vi "Check Cluster Term Type.vi"(8 "Error In (no Error) In":errorcluster, 10 "Element Check In":T1(ring), 11 "Term Type In":T2) -> (0 "Error Out":errorcluster, 3 "Is Good ?":bool, 5 "Elements":i32)   [LabVIEW 2012, in "Scripting Tools.lvlib" / "XNode Support.lvlib"]
doc: "Inspect a terminal to see if it is a cluster with certain characteristics (e.g. all elements the same type, all numeric, all sortable etc)."
uses:
  XNode Support.lvlib
  <vilib>/XNodeSupport/XNodeTermTypeIDPair.ctl
  <vilib>/XNodeSupport/XNodeType.ctl
  <vilib>/XNodeSupport/XNodeString.ctl
  <vilib>/Utility/VariantDataType/VariantType.lvlib
  <vilib>/XNodeSupport/NI_XNodeSupport.lvlib
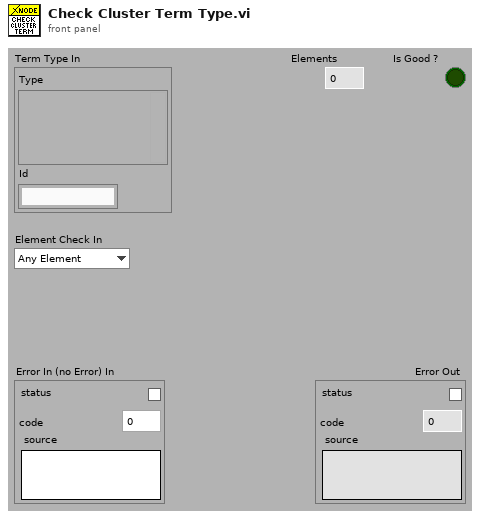
[diagram p1: front panel]
types:
  T1 = enum16{"Any Element", "All Numeric", "All Integer", "All Float", "All Complex", "All Sortable", "Error Cluster", "All the same type"}
  T2 = typedef "NI_XNodeSupport.lvlib/XNodeTermTypeIDPair.ctl" = cluster{"Type":T3, "Id":T4}
  T3 = typedef "NI_XNodeSupport.lvlib/XNodeType.ctl" = variant
  T4 = typedef "NI_XNodeSupport.lvlib/XNodeString.ctl" = string
  T5 = typedef "VariantType.lvlib/Type.ctl" = enum8{"Invalid Type", "Void", "I8", "I16", "I32", "I64", "U8", "U16", "U32", "U64", "Single Float", "Double Float", "Extended Float", "Single Complex", "Double Complex", "Extended Complex", "Enum U8", "Enum U16", "Enum U32", "Enum U64", "Single Float With Unit", "Double Float With Unit", "Extended Float With Unit", "Single Complex with Unit", "Double Complex with Unit", "Extended Complex with Unit", "Boolean", "String", "Path", "Picture", "Tag", "Array", "Cluster", "Variant", "LV Variant", "Waveform", "Timestamp", "Digital Waveform", "Digital Data", "ExpressData", "Refnum", "External Data", "VI", "Poly VI", "LabVIEW Class Instance", "Fixed Point"}
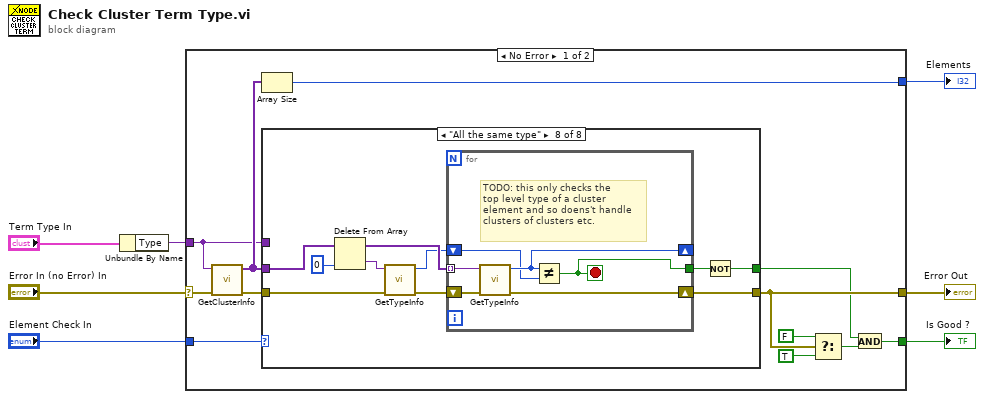
[diagram p0: block diagram]
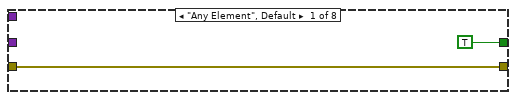
[diagram p2: hidden frame]
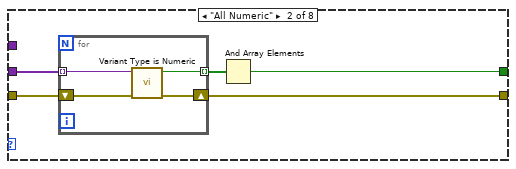
[diagram p3: hidden frame]
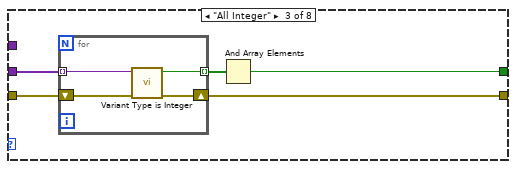
[diagram p4: hidden frame]
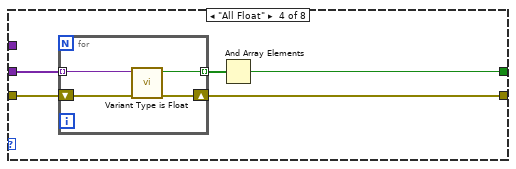
[diagram p5: hidden frame]
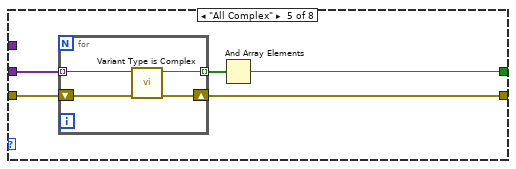
[diagram p6: hidden frame]
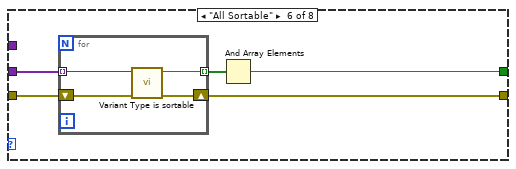
[diagram p7: hidden frame]
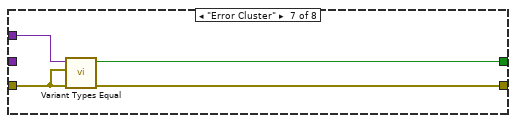
[diagram p8: hidden frame]
diagram:
  n1 = Unbundle By Name("Term Type In") -> ("Type"=w5:T3)
  n2 = case shown="No Error" "Error In (no Error) In" {
    selector: "Error In (no Error) In" -> [w19 w87]
    tunnel: w5 -> [w9 _]
    tunnel: [w18 _] -> w4
    tunnel: "Element Check In" -> [w17 _]
    tunnel: [w15 w87] -> w2
    tunnel: [w11 _] -> w1
    frame No Error {
      n3 = call <vilib>:"GetClusterInfo.vi"("error in (no error)"=w19, "Variant"=w9) -> ("error out"=w16:errorcluster, "Cluster Elements"=w10:variant[])  [unwired: 8 out]
      n4 = Array Size(array=w10) -> (size(s)=w18:i32)
      n5 = case shown="\"All the same type\"" w17 {
        tunnel: w16 -> [w21 w26 w35 w44 w53 w62 w70 w76]
        tunnel: [w21 w25 w34 w43 w52 w61 w68 w73] -> w15
        tunnel: [TRUE w24 w33 w42 w51 w60 w67 w71] -> w12
        tunnel: w10 -> [_ w23 w32 w41 w50 w59 _ w80]
        tunnel: w9 -> [_ _ _ _ _ _ w69 _]
        frame "Any Element", Default {
        }
        frame "All Numeric" {
          n6 = for {
            shift-right: [w27] -> w25
            shift-left: w26 -> [w30]
            tunnel: w23 -> [w29] mode=indexing
            tunnel: [w28] -> w22 mode=indexing
            n7 = call "Variant Type is Numeric.vi"("error in (no error)"=w30, "Type"=w29) -> ("error out"=w27:errorcluster, "Sortable ?"=w28:bool)  [unwired: 8 out]
          }
          n8 = And Array Elements(Boolean array=w22) -> (logical AND=w24:bool)
        }
        frame "All Integer" {
          n9 = for {
            shift-right: [w36] -> w34
            shift-left: w35 -> [w39]
            tunnel: w32 -> [w38] mode=indexing
            tunnel: [w37] -> w31 mode=indexing
            n10 = call "Variant Type is Integer.vi"("error in (no error)"=w39, "Type"=w38) -> ("error out"=w36:errorcluster, "Sortable ?"=w37:bool)  [unwired: 8 out]
          }
          n11 = And Array Elements(Boolean array=w31) -> (logical AND=w33:bool)
        }
        frame "All Float" {
          n12 = for {
            shift-right: [w45] -> w43
            shift-left: w44 -> [w48]
            tunnel: w41 -> [w47] mode=indexing
            tunnel: [w46] -> w40 mode=indexing
            n13 = call "Variant Type is Float.vi"("error in (no error)"=w48, "Type"=w47) -> ("error out"=w45:errorcluster, "Sortable ?"=w46:bool)  [unwired: 8 out]
          }
          n14 = And Array Elements(Boolean array=w40) -> (logical AND=w42:bool)
        }
        frame "All Complex" {
          n15 = for {
            shift-right: [w54] -> w52
            shift-left: w53 -> [w57]
            tunnel: w50 -> [w56] mode=indexing
            tunnel: [w55] -> w49 mode=indexing
            n16 = call "Variant Type is Complex.vi"("error in (no error)"=w57, "Type"=w56) -> ("error out"=w54:errorcluster, "Sortable ?"=w55:bool)  [unwired: 8 out]
          }
          n17 = And Array Elements(Boolean array=w49) -> (logical AND=w51:bool)
        }
        frame "All Sortable" {
          n18 = for {
            shift-right: [w63] -> w61
            shift-left: w62 -> [w66]
            tunnel: w59 -> [w65] mode=indexing
            tunnel: [w64] -> w58 mode=indexing
            n19 = call "Variant Type is sortable.vi"("error in (no error)"=w66, "Type"=w65) -> ("error out"=w63:errorcluster, "Sortable ?"=w64:bool)  [unwired: 8 out]
          }
          n20 = And Array Elements(Boolean array=w58) -> (logical AND=w60:bool)
        }
        frame "Error Cluster" {
          n21 = call "Variant Types Equal.vi"("error in (no error)"=w70, "Type"=w70, "Type to Test"=w69) -> ("error out"=w68:errorcluster, "Same Type"=w67:bool)  [unwired: 7 out]
        }
        frame "All the same type" {
          n22 = Delete From Array(array=w80, index=0) -> (deleted portion=w77:variant, array with subset deleted=w79:variant[])  [unwired: 1 in]
          n23 = call <vilib>:"GetTypeInfo.vi"("error in (no error)"=w76, "Variant"=w77) -> ("error out"=w75:errorcluster, "Type Enum"=w74:T5)  [unwired: 8 out]
          n24 = for {
            tunnel: w79 -> [w86] mode=indexing
            shift-right: [w82] -> w73
            shift-left: w75 -> [w85]
            shift-right: [w84] -> _
            shift-left: w74 -> [w83]
            tunnel: [w81] -> w72
            stop <- w81 stop-if-true
            # "TODO: this only checks the \ntop level type of a cluster\nelement and so doens't handle\nclusters of clusters etc."
            n25 = call <vilib>:"GetTypeInfo.vi"("error in (no error)"=w85, "Variant"=w86) -> ("error out"=w82:errorcluster, "Type Enum"=w84:T5)  [unwired: 8 out]
            n26 = Not Equal?(x=w84, y=w83) -> (x != y?=w81:bool)
          }
          n27 = Not(x=w72) -> (.not. x?=w71:bool)
        }
      }
      n28 = Select(t=FALSE, s=w15, f=TRUE) -> (s? t:f=w13:bool)
      n29 = And(x=w12, y=w13) -> (x .and. y?=w11:bool)
    }
    frame Error {
    }
  }
  "Elements" <- w4
  "Error Out" <- w2
  "Is Good ?" <- w1
